vi "PMD Get Power.vi"(0 "VISA In":refnum<visa-resource-name>, 1 "Wavelength (nm)":dbl=100.0 min=0.0 max=2000.0 step=0.1 format="%.1f", 2 "Timeout (100 ms)":i32=100, 3 "error in":errorcluster) -> (4 "New":bool, 5 "PMD Error":string, 6 "VISA out":refnum<visa-resource-name>, 7 "Readout value":dbl format="%^#_9e", 8 "Readout string":string, 9 "error out":errorcluster)   [LabVIEW 2013]
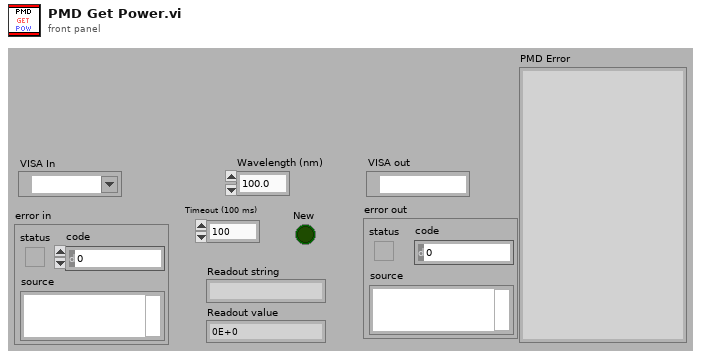
[diagram p1: front panel]
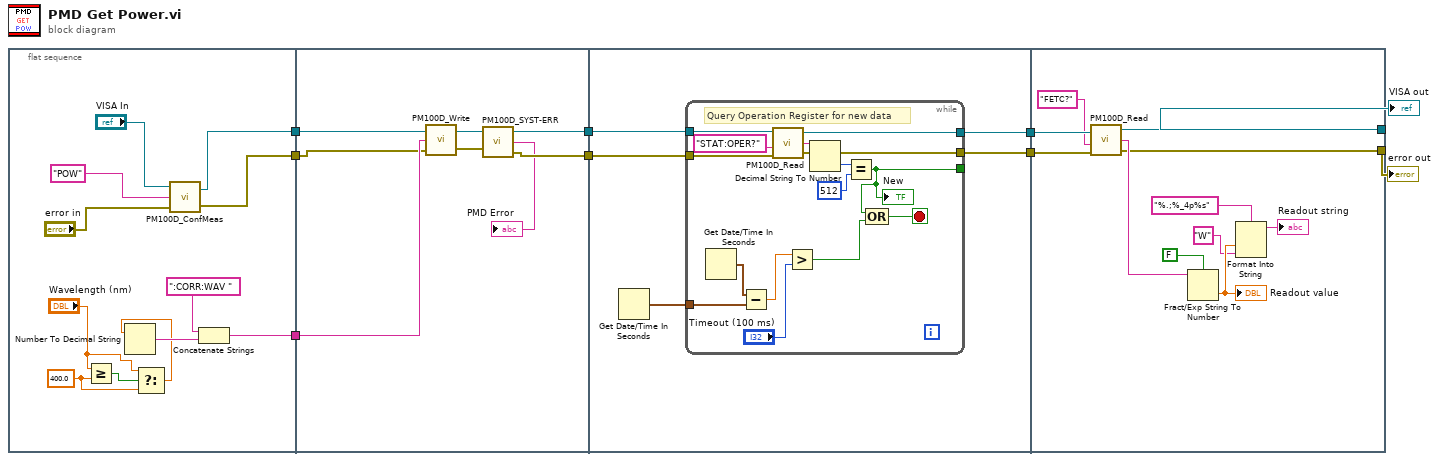
[diagram p0: block diagram]
diagram:
  n1 = flat-sequence {
    tunnel: [w20] -> w5
    tunnel: [w19] -> w3
    tunnel: [w14] -> w1
    tunnel: w5 -> [w28]
    tunnel: [w24] -> w4
    tunnel: w3 -> [w27]
    tunnel: [w23] -> w2
    tunnel: w1 -> [w29]
    tunnel: w4 -> [w34]
    tunnel: w2 -> [w33]
    tunnel: [w31] -> w9
    tunnel: [w30] -> w8
    tunnel: w9 -> [w60]
    tunnel: w8 -> [w59]
    tunnel: [w51] -> w6
    tunnel: [w50] -> w7
    frame #0 {
      w11 = 400.0 ("y")
      n2 = Greater Or Equal?(x="Wavelength (nm)", y=w11) -> (x >= y?=w13:bool)
      n3 = Select(t="Wavelength (nm)", s=w13, f=w11) -> (s? t:f=w10:dbl)
      n4 = Number To Decimal String(number=w10) -> (decimal integer string=w16:string)  [unwired: 1 in]
      n5 = call "PM100D_ConfMeas.vi"("error in"="error in", "Conf:"="POW" ("Command"), "VISA In"="VISA In") -> ("error out"=w19:errorcluster, "dup VISA session"=w20:refnum<visa-resource-name>)
      n6 = Concatenate Strings(":CORR:WAV " ("string"), w16) -> (w14:string)
    }
    frame #1 {
      n7 = call "PM100D_Write.vi"("error in (no error)"=w27, "Command"=w29, "VISA in"=w28) -> ("error out"=w25:errorcluster, "VISA out"=w26:refnum<visa-resource-name>)
      n8 = call "PM100D_SYST-ERR.vi"("error out 2"=w25, "VISA In"=w26) -> ("error out"=w23:errorcluster, "Error"=→"PMD Error":string, "VISA Out"=w24:refnum<visa-resource-name>)  [unwired: 1 in]
    }
    frame #2 {
      n9 = Get Date/Time In Seconds() -> (seconds since 1Jan1904=w32:timestamp)
      n10 = while {
        tunnel: w34 -> [w45]
        tunnel: w33 -> [w44]
        tunnel: [w43] -> w31
        tunnel: [w42] -> w30
        tunnel: [w40] -> _
        tunnel: w32 -> [w38]
        stop <- w41 stop-if-true
        # "Query Operation Register for new data"
        n11 = Get Date/Time In Seconds() -> (seconds since 1Jan1904=w39:timestamp)
        n12 = Subtract(x=w39, y=w38) -> (x-y=w37:dbl)
        n13 = call "PM100D_Read.vi"("error in (no error)"=w44, "Command"="STAT:OPER?", "VISA in"=w45) -> ("error out"=w42:errorcluster, "ReadValue"=w48:string, "VISA out"=w43:refnum<visa-resource-name>)  [unwired: 1 in]
        n14 = Greater?(x=w37, y="Timeout (100 ms)") -> (0:w35:bool)
        n15 = Decimal String To Number(string=w48) -> (number=w47:i32)  [unwired: 2 in, 1 out]
        n16 = Equal?(x=w47, y=512) -> (x = y?=w40:bool)
        "New" <- w40
        n17 = Compound Arithmetic op=OR(w40, w35) -> (w41:bool)
      }
    }
    frame #3 {
      n18 = call "PM100D_Read.vi"("error in (no error)"=w59, "Command"="FETC?", "VISA in"=w60) -> ("error out"=w50:errorcluster, "ReadValue"=w52:string, "VISA out"=w51:refnum<visa-resource-name>)  [unwired: 1 in]
      n19 = Fract/Exp String To Number(use system decimal point (T)=FALSE, string=w52) -> (number=w55:dbl)  [unwired: 2 in, 1 out]
      "Readout value" <- w55
      n20 = Format Into String(format string="%.;%_4p%s", w55, "W") -> (resulting string=→"Readout string":string)  [unwired: 2 in, 1 out]
    }
  }
  "error out" <- w7
  "VISA out" <- w6
